vi "Climb_Set.vi"   [LabVIEW 2019]
uses:
  Globals/Climb_Globals.vi
types:
  T1 = enum16{"No-Op", "Extending", "Clamping", "Balancing", "Manual_Control"}
  T2 = typedef "Climb_Cluster.ctl" = cluster{"Control_State":enum16{"No-Op", "Extending", "Clamping", "Balancing", "Manual_Control"}, "Extend_Climber?":bool, "Clamp?":bool, "Balance?":bool, "Manual_Control?":bool, "Joint_Throttle":dbl, "LeadScrew_Throttle":dbl}
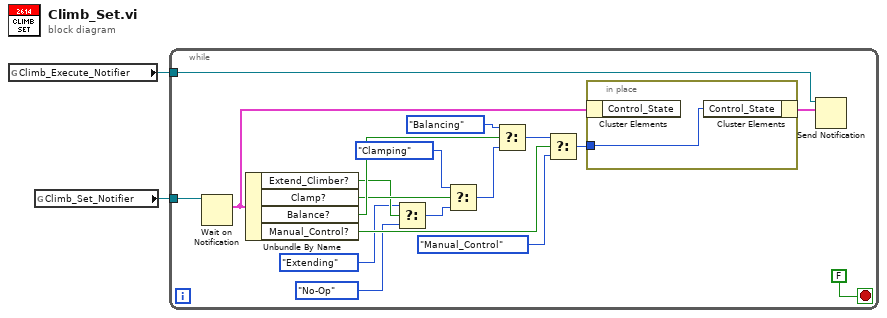
[diagram p0: block diagram]
diagram:
  n1 = global read "Climb_Globals.vi" "Climb_Execute_Notifier"() -> (w1:refnum<notifier>)
  n2 = global read "Climb_Globals.vi" "Climb_Set_Notifier"() -> (w2:refnum<notifier>)
  n3 = while {
    tunnel: w2 -> [w20]
    tunnel: w1 -> [w19]
    stop <- FALSE stop-if-true
    n4 = Wait on Notification(notifier=w20) -> (notification=w17:T2)  [unwired: 3 in, 3 out]
    n5 = Unbundle By Name(w17) -> ("Extend_Climber?"=w11:bool, "Clamp?"=w12:bool, "Balance?"=w14:bool, "Manual_Control?"=w16:bool)
    n6 = Select(t=T1."Extending" ("Control_State"), s=w11, f=T1."No-Op" ("Control_State")) -> (s? t:f=w10:T1)
    n7 = Select(t=T1."Clamping" ("Control_State"), s=w12, f=w10) -> (s? t:f=w13:T1)
    n8 = Select(t=T1."Balancing" ("Control_State"), s=w14, f=w13) -> (s? t:f=w15:T1)
    n9 = Select(t=w15, s=w16, f=T1."Manual_Control" ("Control_State")) -> (s? t:f=w9:T1)
    n10 = in-place {
      in-place-border: w9 -> [w21]
      n11 = in-place-cluster #1(w17) -> ()  [unwired: 1 out]
      n12 = in-place-cluster #1("Control_State"=w21) -> (w8:T2)
    }
    n13 = Send Notification(notification=w8, notifier=w19) -> ()  [unwired: 1 in, 2 out]
  }
